vi "ActionVIOnSave.vi"(8 "error in (no error)":errorcluster, 11 "Device Item Ref in":T1 format="%.0x") -> (0 "error out":errorcluster, 3 "Device Item Ref out":T1 format="%.0x")   [LabVIEW 2019, in "Diagnostics Addon System Explorer.lvlib"]
uses:
  Diagnostics Addon System Explorer.lvlib
  <vilib>/NI VeriStand/Custom Device API/Custom Device Item Ref.ctl
  Types/FG.Action.ctl
  Addon Shared/SubVIs/Constants.vi
  <vilib>/NI VeriStand/Custom Device Tools/Custom Device Utility Library/NI VeriStand - Search for Item by GUID.vi
  <vilib>/NI VeriStand/Custom Device Tools/Custom Device Utility Library/NI VeriStand - Search for All Items by GUID.vi
  <vilib>/NI/NI VeriStand Advanced SysDef API/SysDef API/SysDef.Property.Set.vi
  <vilib>/NI/NI VeriStand Advanced SysDef API/_SubVIs/SysDef.Property.Set.U32.vi
  <vilib>/NI VeriStand/Custom Device API/NI VeriStand - Get Item Property.vi
  <vilib>/NI VeriStand/Custom Device API/Get Item Property (U32).vi
  <vilib>/NI/NI VeriStand Advanced SysDef API/_SubVIs/SysDef.Property.Set.U32.Array.vi
  <vilib>/NI VeriStand/Custom Device API/Get Item Property (U32 Array).vi
  <vilib>/NI VeriStand/Custom Device Tools/Custom Device Utility Library/Custom Device Utility Library.lvlib
  Addon Shared/Diagnostics Addon Shared.lvlib
  <vilib>/NI VeriStand/Custom Device API/Custom Device API.lvlib
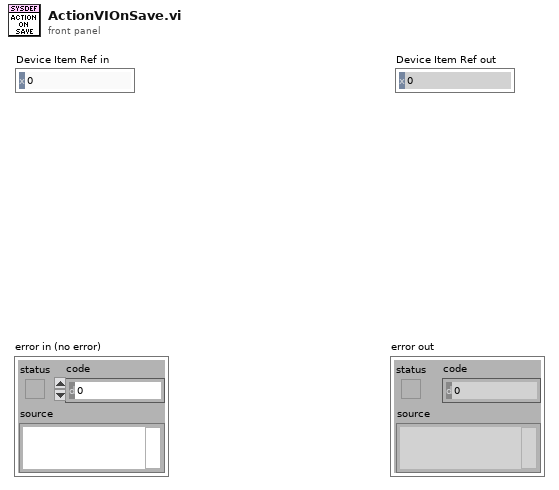
[diagram p1: front panel]
types:
  T1 = typedef "Custom Device API.lvlib/Custom Device Item Ref.ctl" = u64
  T2 = typedef "Diagnostics Addon System Explorer.lvlib/FG.Action.ctl" = enum16{"Get", "Set"}
  T3 = typedef "Diagnostics Addon Shared.lvlib/DPID.ctl" = cluster{"DPID ID":u8, "Speed":T4, "PIDs":u16[]}
  T4 = typedef "Diagnostics Addon Shared.lvlib/DPID.Rate.ctl" = enum16{"Slow", "Medium", "Fast"}
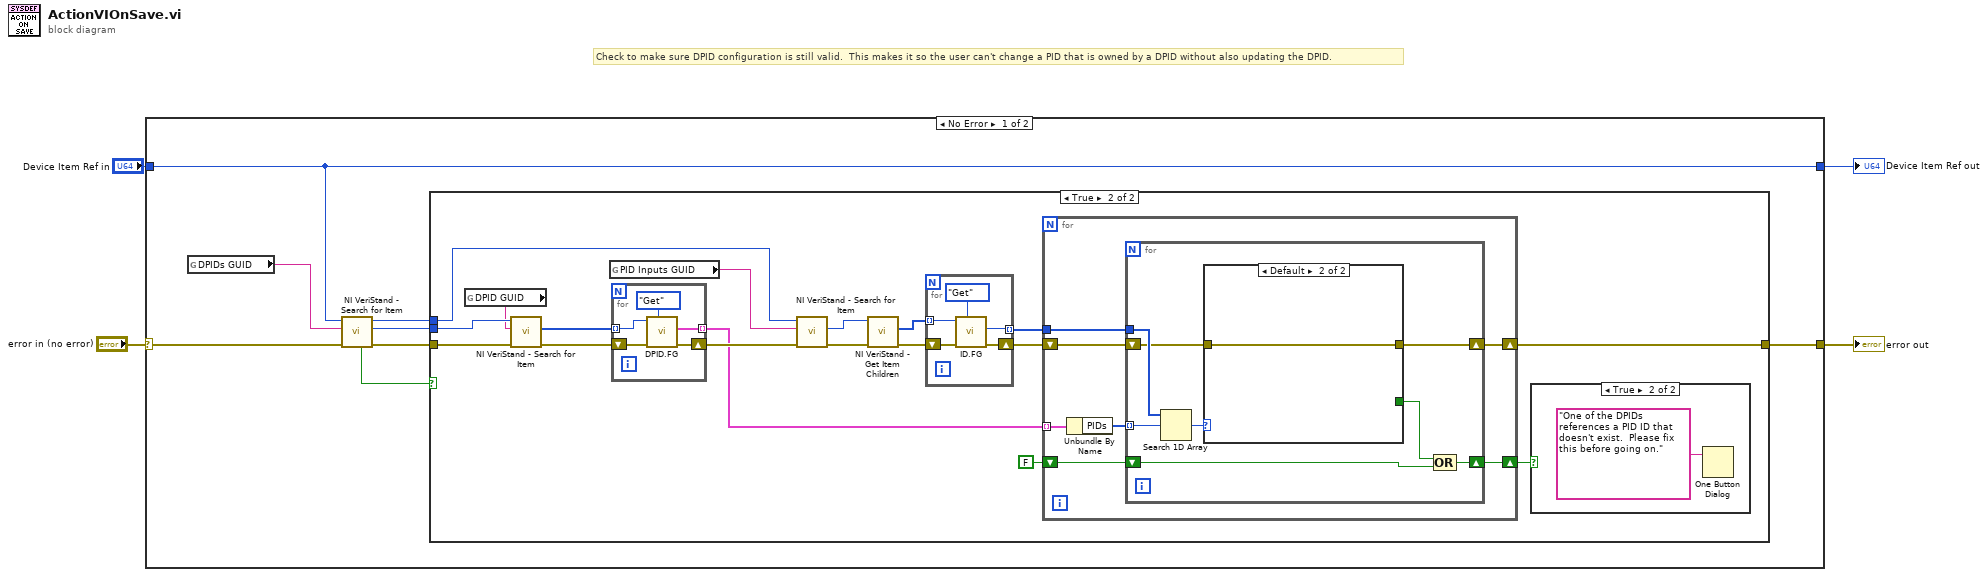
[diagram p0: block diagram]
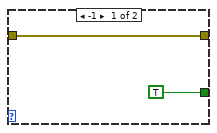
[diagram p4: hidden frame]
diagram:
  # "Check to make sure DPID configuration is still valid.  This makes it so the user can't change a PID that is owned by a DPID without also updating the DPID."
  n1 = case shown="No Error" "error in (no error)" {
    selector: "error in (no error)" -> [w12 w62]
    tunnel: [w5 w62] -> w3
    tunnel: "Device Item Ref in" -> [w6 w61]
    tunnel: [w6 w61] -> w1
    frame No Error {
      n2 = global read "Constants.vi" "DPIDs GUID"() -> (w11:string)
      n3 = call-poly <vilib>:"NI VeriStand - Search for Item.vi"("error in"=w12, "Item GUID"=w11, "Section Ref in"=w6) -> ("error out"=w8:errorcluster, "Item Ref"=w9:T1, "Section Ref out"=w7:T1, "Found"=w10:bool)  [unwired: 5 in]
      n4 = case shown="True" w10 {
        tunnel: w9 -> [_ w30]
        tunnel: w8 -> [w13 w31]
        tunnel: [w13 w17] -> w5
        tunnel: w7 -> [_ w16]
        frame False {
        }
        frame True {
          n5 = global read "Constants.vi" "DPID GUID"() -> (w14:string)
          n6 = call-poly <vilib>:"NI VeriStand - Search for Item.vi"("error in"=w31, "Item GUID"=w14, "Section Ref in"=w30) -> ("error out"=w29:errorcluster, "Item Refs"=w28:T1[])  [unwired: 5 in, 2 out]
          n7 = global read "Constants.vi" "PID Inputs GUID"() -> (w26:string)
          n8 = for {
            tunnel: w28 -> [w59] mode=indexing
            shift-right: [w58] -> w27
            shift-left: w29 -> [w60]
            tunnel: [w57] -> w20 mode=indexing
            n9 = call "DPID.FG.vi"("Action"=FG.Action."Get", "error in (no error)"=w60, "Device Item Ref in"=w59) -> ("error out"=w58:errorcluster, "DPID"=w57:T3)  [unwired: 6 in, 1 out]
          }
          n10 = call-poly <vilib>:"NI VeriStand - Search for Item.vi"("error in"=w27, "Item GUID"=w26, "Section Ref in"=w16) -> ("error out"=w25:errorcluster, "Item Ref"=w24:T1)  [unwired: 5 in, 2 out]
          n11 = call <vilib>:"NI VeriStand - Get Item Children.vi"("error in (no error)"=w25, "Item Ref in"=w24) -> ("error out"=w23:errorcluster, "Child Refs"=w22:T1[])  [unwired: 6 in, 2 out]
          n12 = for {
            tunnel: w22 -> [w55] mode=indexing
            shift-right: [w53] -> w19
            shift-left: w23 -> [w54]
            tunnel: [w52] -> w21 mode=indexing
            n13 = call "ID.FG.vi"("Action"=FG.Action."Get", "error in (no error)"=w54, "Device Item Ref in"=w55) -> ("error out"=w53:errorcluster, "ID"=w52:u32)  [unwired: 6 in, 1 out]
          }
          n14 = for {
            tunnel: w21 -> [w39]
            tunnel: w20 -> [w38] mode=indexing
            shift-right: [w33] -> w17
            shift-left: w19 -> [w36]
            shift-right: [w34] -> w15
            shift-left: FALSE -> [w35]
            n15 = Unbundle By Name(w38) -> ("PIDs"=w37:u16[])
            n16 = for {
              tunnel: w37 -> [w43] mode=indexing
              shift-right: [w44] -> w33
              shift-left: w36 -> [w45]
              tunnel: w39 -> [w47]
              shift-right: [w41] -> w34
              shift-left: w35 -> [w40]
              n17 = Search 1D Array(1D array=w47, element=w43) -> (index of element=w46:i32)  [unwired: 1 in]
              n18 = case shown="Default" w46 {
                tunnel: [w49 w50] -> w44
                tunnel: w45 -> [w49 w50]
                tunnel: [TRUE _] -> w42
                frame -1 {
                }
                frame Default {
                }
              }
              n19 = Compound Arithmetic op=OR(w42, w40) -> (w41:bool)
            }
          }
          n20 = case shown="True" w15 {
            frame False {
            }
            frame True {
              n21 = One Button Dialog(message="One of the DPIDs references a PID ID that doesn't exist.  Please fix this before going on.") -> ()  [unwired: 1 in, 1 out]
            }
          }
        }
      }
    }
    frame Error {
    }
  }
  "error out" <- w3
  "Device Item Ref out" <- w1
